vi "Read Image Msg.vi"(8 "error in (no error)":errorcluster, 11 "Image Acquisition in":refnum<class "Image Acquisition.lvclass">) -> (0 "error out":errorcluster, 2 "Image Acquisition.lvlib:Image Msg.lvclass":refnum<class "Image Msg.lvclass">, 3 "Image Acquisition out":refnum<class "Image Acquisition.lvclass">)   [LabVIEW 2016, in "Image Acquisition.lvlib" / "Image Acquisition.lvclass"]
uses:
  Image Acquisition.lvclass
  Image Acquisition Messages/Image Msg/Image Msg.lvclass
  Image Acquisition.lvclass/Image Acquisition.ctl
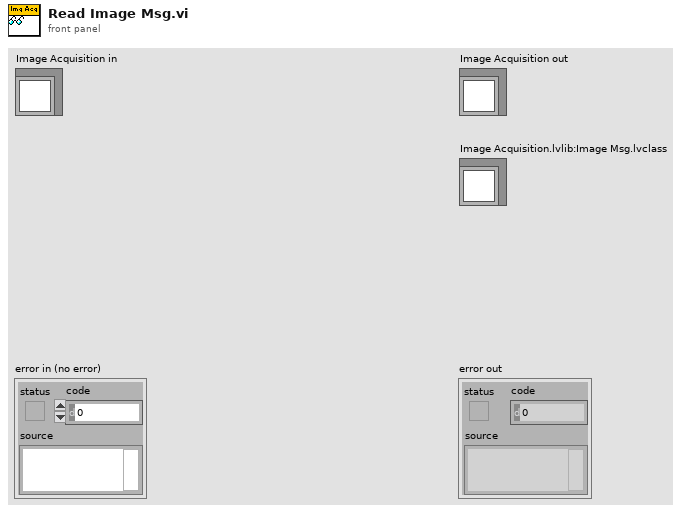
[diagram p1: front panel]
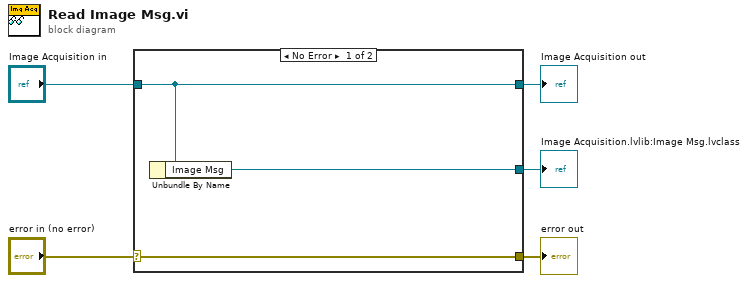
[diagram p0: block diagram]
diagram:
  n1 = case shown="No Error" "error in (no error)" {
    selector: "error in (no error)" -> [w8 w9]
    tunnel: [w8 w9] -> w4
    tunnel: [w7 w10] -> w2
    tunnel: "Image Acquisition in" -> [w7 w10]
    tunnel: [w6 _] -> w1
    frame No Error {
      n2 = Unbundle By Name(w7) -> ("Image Msg"=w6:refnum<class "Image Msg.lvclass">)
    }
    frame Error {
    }
  }
  "error out" <- w4
  "Image Acquisition out" <- w2
  "Image Acquisition.lvlib:Image Msg.lvclass" <- w1
